vi "Single Sensor.vi"() -> ()   [LabVIEW 2012]
uses:
  <vilib>/rvi/interface/nirviOpenFPGA/nirviOpenFPGA.xnode
  <vilib>/rvi/interface/nirviReadWriteControl/nirviReadWriteControl.xnode
  <vilib>/rvi/interface/Simulation/niFpgaSimulationCallBeginRW.vi
  <vilib>/rvi/errors/niLvFpgaAdjustHostInterfaceError.vi
panel:
  out "ModA/AI0":fxp<+/-,26,5>
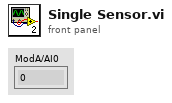
[diagram p1: front panel]
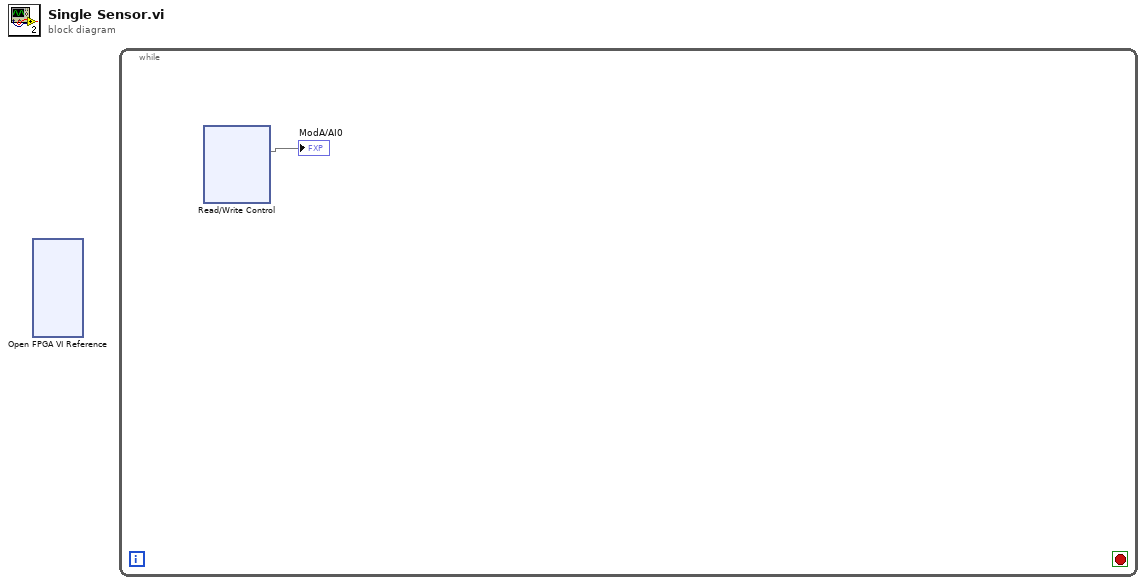
[diagram p0: block diagram]
diagram:
  n1 = xnode "Open FPGA VI Reference"() -> ()  [unwired: 2 in, 2 out]
  n2 = while {
    stop <- _ stop-if-true
    n3 = xnode "Read/Write Control"() -> ("ModA/AI0"=→"ModA/AI0")  [unwired: 2 in, 5 out]
  }
